vi "IO nucleus.vi"(2 "cf":dbl=3.1206440978827352) -> (0 "cfs":dbl[](array[numeric])=[0.2996515278306188, 0.0])   [LabVIEW 2016]
panel:
  in  "cf gain":dbl=0.01
  out "Climbing Fibers":cluster{dbl, "f":dbl, "f":dbl}(graph)
  out "Right":dbl
  out "Left":dbl=0.2996515278306188
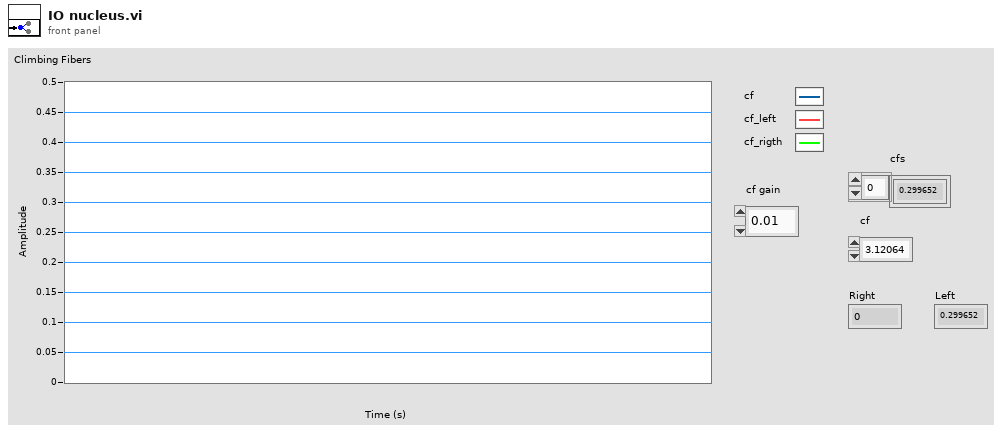
[diagram p1: front panel]
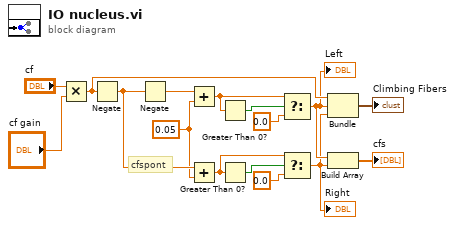
[diagram p0: block diagram]
diagram:
  w3 = 0.05 ("cf spont")
  # "cfspont"
  n1 = Multiply(x="cf", y="cf gain") -> (x*y=w6:dbl)
  n2 = Negate(x=w6) -> (-x=w9:dbl)
  n3 = Negate(x=w9) -> (-x=w15:dbl)
  n4 = Add(x=w15, y=w3) -> (x+y=w16:dbl)
  n5 = Add(x=w9, y=w3) -> (x+y=w10:dbl)
  n6 = Greater Than 0?(x=w16) -> (x > 0?=w14:bool)
  n7 = Greater Than 0?(x=w10) -> (x > 0?=w11:bool)
  n8 = Select(t=w16, s=w14, f=0.0) -> (s? t:f=w4:dbl)
  "Left" <- w4
  n9 = Select(t=w10, s=w11, f=0.0) -> (s? t:f=w1:dbl)
  "Right" <- w1
  n10 = Bundle(w6, "f"=w4, "f"=w1) -> (→"Climbing Fibers":cluster{dbl, "f":dbl, "f":dbl})  [unwired: 1 in]
  n11 = Build Array(w4, w1) -> (→"cfs":dbl[])
